vi "period-duty-time-high-low.vi"(9 "Duty Cycle":dbl, 10 "Period (Seconds)":dbl) -> (0 "Time High (Seconds)":dbl, 1 "Time Low (Seconds)":dbl, 3 "delaytimes mS":cluster{"low":dbl, "high":dbl}, 4 "Duty %":dbl)   [LabVIEW 2021]
panel:
  out "Time Low mS":dbl
  out "Time High mS":dbl
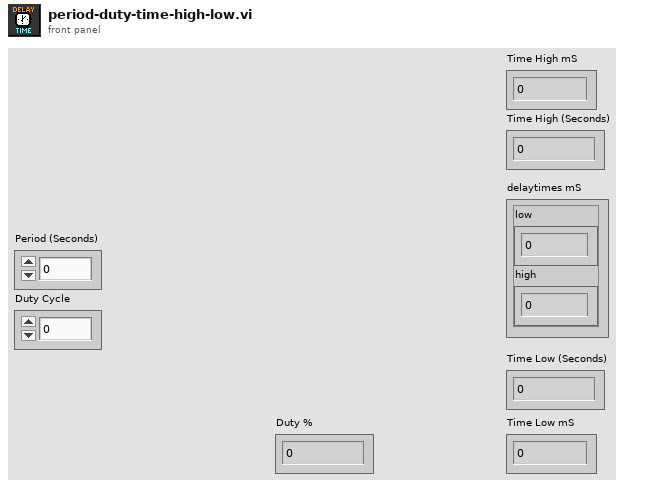
[diagram p1: front panel]
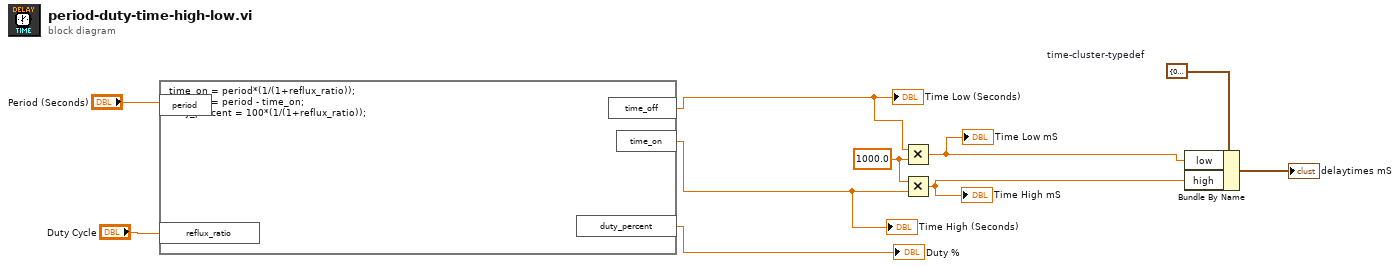
[diagram p0: block diagram]
diagram:
  w1 = 1000.0 ("y")
  w9 = cluster{"low":dbl, "high":dbl} {"low"=0.0, "high"=0.0}  # time-cluster-typedef
  n1 = formula code="time_on = period*(1/(1+reflux_ratio));\ntime_off = period - time_on;\nduty_percent = 100*(1/(1+reflux_ratio));"("period"="Period (Seconds)", "reflux_ratio"="Duty Cycle") -> ("time_on"=w3:dbl, "time_off"=w6:dbl, "duty_percent"=→"Duty %":dbl)
  "Time High (Seconds)" <- w3
  "Time Low (Seconds)" <- w6
  n2 = Multiply(x=w6, y=w1) -> (x*y=w8:dbl)
  "Time Low mS" <- w8
  n3 = Multiply(x=w1, y=w3) -> (x*y=w7:dbl)
  "Time High mS" <- w7
  n4 = Bundle By Name(cluster=w9, "low"=w8, "high"=w7) -> (→"delaytimes mS":cluster{"low":dbl, "high":dbl})
